vi "SS2 Live_Download Multiple SS2 Images_v4.vi"(8 "Error In":errorcluster, 9 "# 8-bit Images (1)":i32=1, 10 "Buffer Size (#8-bit Images)":i32, 11 "SS2 Live Internal Variables":T1={"okCFrontPanelDevices Refnum"=refnum, "Device Refnum"=refnum, "Display Image"=refnum, "# Live Images"=0, "relative s"=0.0, "# Image Sets"=0, "Message"="", "Current Image Set"=0, "# Datasets"=0, "Current Dataset"=0, "Live Mode"=FALSE, "Recording Mode"=FALSE, "Record Button"=refnum, "Live Button"=refnum, "SS2 Live Gate Data Q Name"="SS2 Live Gate Data Q", "Discard First Image"=FALSE, "Image Information"={"Save ROI Only"=FALSE, "Left"=0, "Top"=0, "Right"=0, "Bottom"=0, "Use Current ROI"=FALSE}, "Image Binning Options"={"Use Image Binning"=FALSE, "X Bin"=1, "Y Bin"=1}, "FPGA Serial Number"="", "PCB Version"=enum."PCB 1"} {"Image Binning Options"."Y Bin" min=1; "Image Binning Options"."X Bin" min=1}) -> (0 "Error Out":errorcluster, 3 "SS2 Live Internal Variables":T1={"okCFrontPanelDevices Refnum"=refnum, "Device Refnum"=refnum, "Display Image"=refnum, "# Live Images"=0, "relative s"=0.0, "# Image Sets"=0, "Message"="", "Current Image Set"=0, "# Datasets"=0, "Current Dataset"=0, "Live Mode"=FALSE, "Recording Mode"=FALSE, "Record Button"=refnum, "Live Button"=refnum, "SS2 Live Gate Data Q Name"="SS2 Live Gate Data Q", "Discard First Image"=FALSE, "Image Information"={"Save ROI Only"=FALSE, "Left"=0, "Top"=0, "Right"=0, "Bottom"=0, "Use Current ROI"=FALSE}, "Image Binning Options"={"Use Image Binning"=FALSE, "X Bin"=1, "Y Bin"=1}, "FPGA Serial Number"="", "PCB Version"=enum."PCB 1"} {"Image Binning Options"."Y Bin" min=1; "Image Binning Options"."X Bin" min=1})   [LabVIEW 2019]
uses:
  SS2 Live Internal Variables.ctl
  C:/UCLA Thinkpad Google Drive/LabVIEW 2019 SP1/builds/SS2 Live Distribution/Opal Kelly/C# Wrapper/libFrontPanel-csharp.dll
  Opal Kelly/C# Wrapper/libFrontPanel-csharp.dll
  <vilib>/vision/Image Controls.llb/IMAQ Image.ctl
  SS2 Live_Image ROI Information.ctl
  Phasor/Image Binning Options.ctl
  SS2 DAQ PCB Version.ctl
  <vilib>/Utility/High Resolution Relative Seconds.vi
  <vilib>/Utility/error.llb/Error Cluster From Error Code.vi
  <vilib>/ErrorRing/Error Ring.xnode
  Opal Kelly/C# Wrapper/okFrontPanelC#Wrapper.lvlib
  Notebook/Notebook.lvlib
  Rich Text Box/Rich Text Box.lvlib
panel:
  out "ReadFromBlockPipeout Error":errorcluster
  out "Activate Trigger Error Out":errorcluster
  out "Timeout error":errorcluster
  out "CPU/8-bit Gate":dbl
  in  "Discard First Image":bool
  in  "Block Size":i32=-1
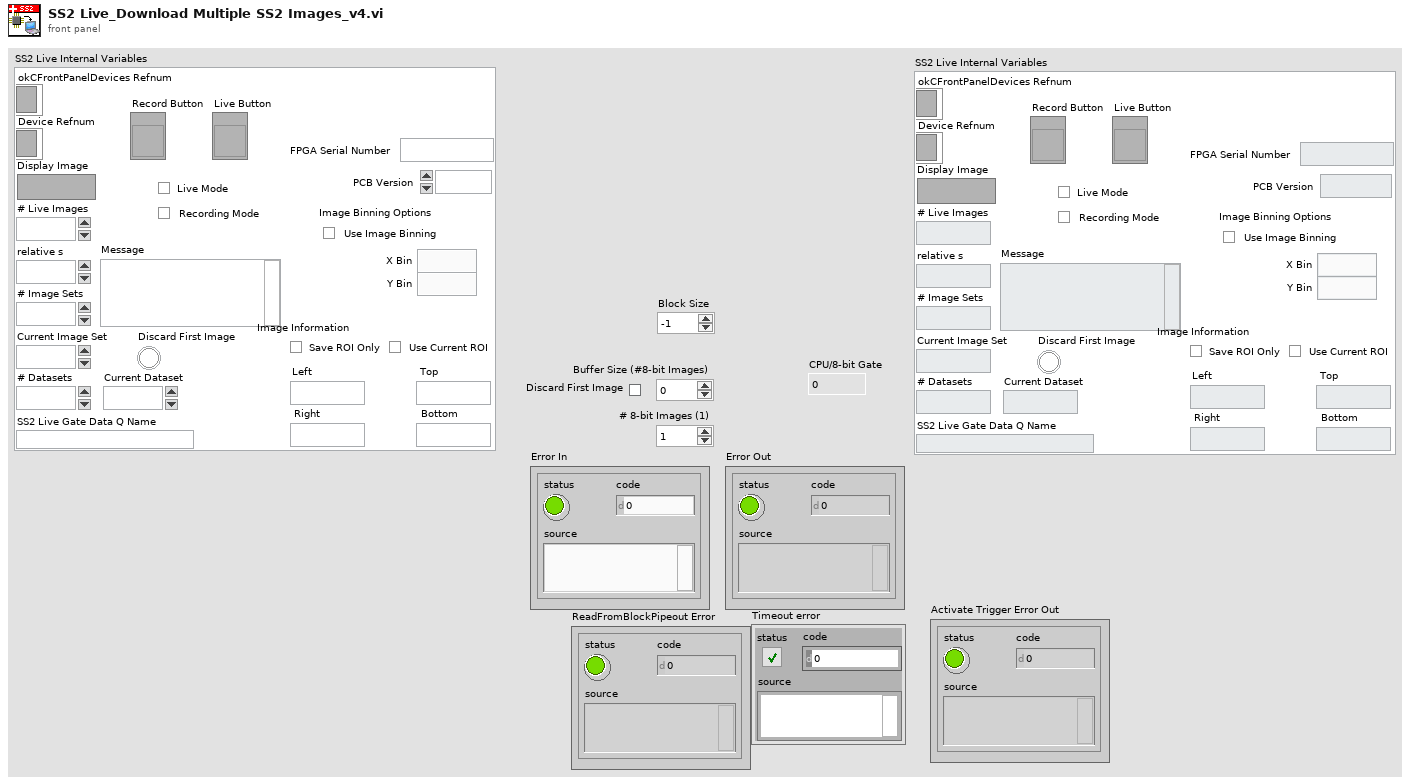
[diagram p1: front panel]
types:
  T1 = typedef "SS2 Live Internal Variables.ctl" = cluster{"okCFrontPanelDevices Refnum":refnum<k24>, "Device Refnum":refnum<k24>, "Display Image":T2, "# Live Images":i32, "relative s":dbl, "# Image Sets":i32, "Message":string, "Current Image Set":i32, "# Datasets":i32, "Current Dataset":i32, "Live Mode":bool, "Recording Mode":bool, "Record Button":refnum<vi>, "Live Button":refnum<vi>, "SS2 Live Gate Data Q Name":string, "Discard First Image":bool, "Image Information":T3, "Image Binning Options":T4, "FPGA Serial Number":string, "PCB Version":T5}
  T2 = typedef "IMAQ Image.ctl" = refnum<image>
  T3 = typedef "SS2 Live_Image ROI Information.ctl" = cluster{"Save ROI Only":bool, "Left":u16, "Top":u16, "Right":u16, "Bottom":u16, "Use Current ROI":bool}
  T4 = typedef "Image Binning Options.ctl" = cluster{"Use Image Binning":bool, "X Bin":i32, "Y Bin":i32}
  T5 = typedef "SS2 DAQ PCB Version.ctl" = enum16{"unknown", "PCB 1", "PCB 2"}
  T6 = typedef "Rich Text Box.lvlib/Text Formatting.ctl" = cluster{"Font":string, "Text Color":T7, "Text Background Color":T7, "Text Style":enum16{"Regular", "Bold", "Italic", "Underline", "Strikeout"}, "Font Size (Points)":dbl, "Text Alignment":i32}
  T7 = typedef "Rich Text Box.lvlib/Text Colors.ctl" = enum16{"Unchanged", "Black", "Blue", "Gray", "Green", "Red", "White"}
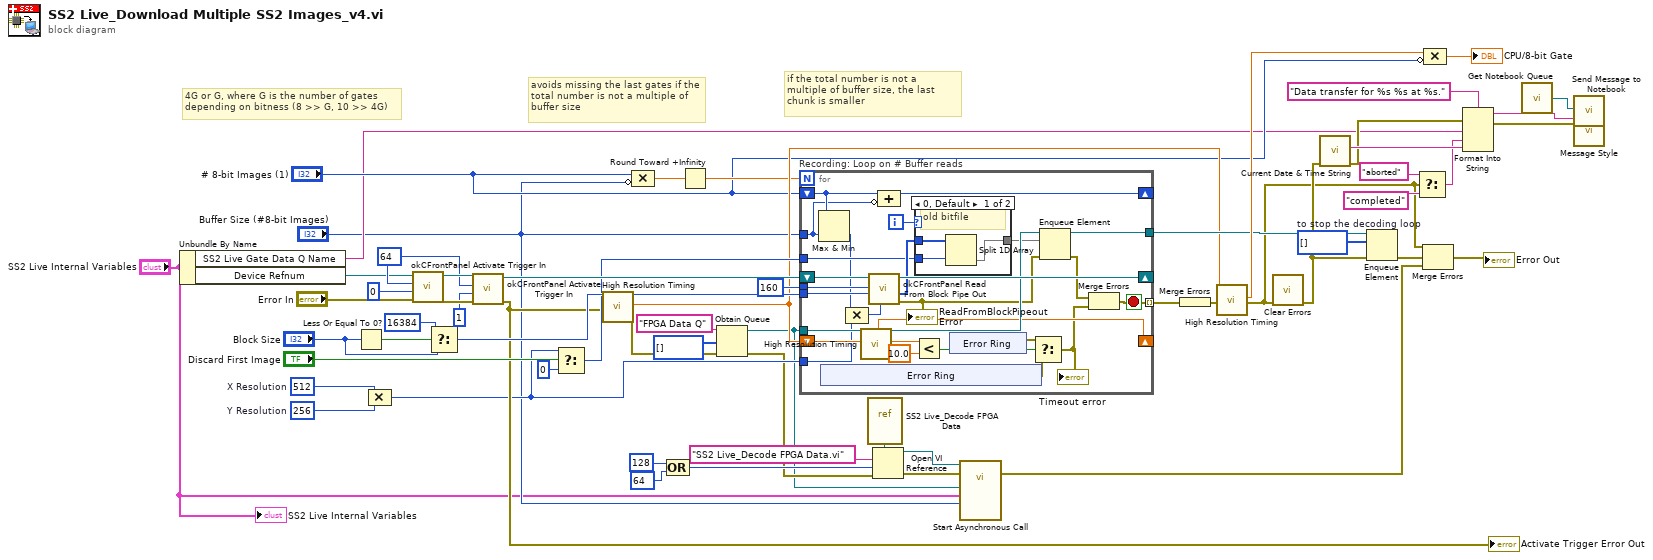
[diagram p0: block diagram]
diagram:
  w42 = u8[] []  # to stop the decoding loop
  w25 = 256  # Y Resolution
  w53 = 512  # X Resolution
  w58 = 64 ("Endpoint Addr")
  # "if the total number is not a multiple of buffer size, the last chunk is smaller"
  # "avoids missing the last gates if the total number is not a multiple of buffer size"
  # "4G or G, where G is the number of gates\ndepending on bitness (8 >> G, 10 >> 4G)"
  n1 = Unbundle By Name("SS2 Live Internal Variables") -> ("SS2 Live Gate Data Q Name"=w20:string, "Device Refnum"=w24:refnum<k24>)
  n2 = Less Or Equal To 0?(x="Block Size") -> (x <= 0?=w56:bool)
  n3 = Compound Arithmetic op=MULTIPLY(w53, w25) -> (w18:i32)
  n4 = call "okCFrontPanel Activate Trigger In.vi"("Error In"="Error In", "Bit"=0, "Endpoint Addr"=w58, "okCFrontPanel Refnum"=w24) -> ("Error Out"=w60:errorcluster, "okCFrontPanel Refnum"=w59:refnum<k24>)  [unwired: 6 in]
  n5 = Select(t=16384, s=w56, f="Block Size") -> (s? t:f=w46:i32)
  n6 = call "okCFrontPanel Activate Trigger In.vi"("Error In"=w60, "Bit"=1, "Endpoint Addr"=w58, "okCFrontPanel Refnum"=w59) -> ("Error Out"=w19:errorcluster, "okCFrontPanel Refnum"=w47:refnum<k24>)  [unwired: 6 in]
  "Activate Trigger Error Out" <- w19
  n7 = Select(t=w18, s="Discard First Image", f=0) -> (s? t:f=w45:i32)
  n8 = call "High Resolution Timing.vi"("Error In"=w19) -> ("elapsed (relative) seconds"=w37:dbl, "Error Out"=w17:errorcluster)  [unwired: 16 in, 1 out]
  n9 = Compound Arithmetic op=MULTIPLY("# 8-bit Images (1)", invert "Buffer Size (#8-bit Images)") -> (w31:dbl)
  n10 = Compound Arithmetic op=OR(128 ("options"), 64 ("options")) -> (w11:i32)
  n11 = Round Toward +Infinity(x=w31) -> (ceil(x): smallest int >= x=w32:dbl)
  n12 = Obtain Queue(name (unnamed)="FPGA Data Q", element data type=u8[] [] ("BYTEARRAY"), error in (no error)=w17) -> (queue out=w6:refnum<queue>, error out=w7:errorcluster)  [unwired: 2 in, 1 out]
  n13 = for "Recording: Loop on # Buffer reads" {
    N: w32 -> [_]
    tunnel: 160 ("Endpoint Addr") -> [w87]
    shift-right: [w85] -> _
    shift-left: w47 -> [w86]
    tunnel: w46 -> [w82]
    tunnel: w45 -> [w69]
    tunnel: w6 -> [w81]
    tunnel: [w62] -> w41 mode=indexing
    tunnel: [w77] -> w38
    shift-right: [w73] -> _
    shift-left: w37 -> [w76]
    shift-right: [w68] -> _
    shift-left: "# 8-bit Images (1)" -> [w67]
    tunnel: "Buffer Size (#8-bit Images)" -> [w66]
    tunnel: w18 -> [w64]
    i -> [w83]
    stop <- w62 stop-if-true
    n14 = Max & Min(x=w67, y=w66) -> (min(x,y)=w65:i32)  [unwired: 1 out]
    n15 = xnode "Error Ring"() -> ("error out"=w71:errorcluster)
    n16 = Compound Arithmetic op=MULTIPLY(w65, w64) -> (w63:i32)
    n17 = call "High Resolution Timing.vi"("relative seconds (NaN)"=w76) -> ("relative seconds"=w73:dbl, "elapsed (relative) seconds"=w75:dbl)  [unwired: 16 in, 1 out]
    n18 = call "okCFrontPanel Read From Block Pipe Out.vi"("Length"=w63, "Block Size"=w82, "Endpoint Addr"=w87, "okCFrontPanel Refnum"=w86) -> ("Error Out"=w79:errorcluster, "BYTEARRAY"=w84:u8[], "okCFrontPanel Refnum"=w85:refnum<k24>)  [unwired: 5 in]
    "ReadFromBlockPipeout Error" <- w79
    n19 = Compound Arithmetic op=ADD(w67, invert w66) -> (w68:i32)
    n20 = Less?(x=w75, y=10.0) -> (x < y?=w72:bool)
    n21 = case shown="0, Default" w83 {
      tunnel: w84 -> [w95 w96]
      tunnel: w69 -> [w94 _]
      tunnel: [w93 w96] -> w80
      frame 0, Default {
        # "old bitfile"
        n22 = Split 1D Array(array=w95, index=w94) -> (second subarray=w93:u8[])  [unwired: 1 out]
      }
      frame 1 {
      }
    }
    n23 = xnode "Error Ring"() -> ("error out"=w70:errorcluster)
    n24 = Select(t=w70, s=w72, f=w71) -> (s? t:f=w61:errorcluster)
    "Timeout error" <- w61
    n25 = Enqueue Element(queue=w81, element=w80, error in (no error)=w79) -> (queue out=w77:refnum<queue>, error out=w78:errorcluster)  [unwired: 1 in, 1 out]
    n26 = Merge Errors(w78, w61) -> (w62:errorcluster)
  }
  n27 = vi-ref "SS2 Live_Decode FPGA Data.vi"() -> (w10:refnum<vi>)
  n28 = Open VI Reference(type specifier VI Refnum (for type only)=w10, vi path="SS2 Live_Decode FPGA Data.vi" ("Notebook Message"), options=w11, error in (no error)=w7) -> (vi reference=w9:refnum<vi>, error out=w8:errorcluster)  [unwired: 2 in]
  n29 = call-by-ref "Start Asynchronous Call"(reference=w9, error in=w8, "Buffer Size (#8-bit Images)"="Buffer Size (#8-bit Images)", "SS2 Live Internal Variables"="SS2 Live Internal Variables", "FPGA Data Q"=w6) -> (error out=w2:errorcluster)  [unwired: 9 in, 1 out]
  n30 = Merge Errors(w41) -> (w39:errorcluster)
  n31 = call "High Resolution Timing.vi"("relative seconds (NaN)"=w37, "Error In"=w39) -> ("elapsed (relative) seconds"=w40:dbl, "Error Out"=w1:errorcluster)  [unwired: 15 in, 1 out]
  n32 = call <vilib>:"Clear Errors.vi"("error in (no error)"=w1) -> ("error out"=w16:errorcluster)  [unwired: 5 in, 1 out]
  n33 = call "Current Date & Time String.vi"("Error In"=w16) -> ("Error Out"=w27:errorcluster, "time string"=w28:string)  [unwired: 8 in, 1 out]
  n34 = Enqueue Element(queue=w38, element=w42, error in (no error)=w16) -> (error out=w15:errorcluster)  [unwired: 1 in, 2 out]
  n35 = Select(t="aborted" ("input 2"), s=w1, f="completed" ("input 2")) -> (s? t:f=w21:string)
  n36 = Merge Errors(w1, w15, w2) -> (→"Error Out":errorcluster)
  n37 = Compound Arithmetic op=MULTIPLY(w40, invert "# 8-bit Images (1)") -> (→"CPU/8-bit Gate":dbl)
  n38 = Format Into String(format string="Data transfer for %s %s at %s.", error in=w27, w20, w21, w28) -> (resulting string=w34:string, error out=w29:errorcluster)  [unwired: 1 in]
  n39 = call "Get Notebook Queue.vi"() -> ("Notebook Queue"=w26:refnum<queue>)  [unwired: 9 in]
  n40 = call "Message Style.vi"() -> ("Message Formatting"=w36:T6)
  n41 = call "Send Message to Notebook.vi"("Notebook Queue"=w26, "Message"=w34, "Error In"=w29, "Text Formatting"=w36) -> ()  [unwired: 15 in, 1 out]
  "SS2 Live Internal Variables" <- "SS2 Live Internal Variables"
